vi "曲线模型计算.vi"(11 "曲线模型":T2={"标液浓度1"=0.0, "测量吸光度1"=0.0, "样品1启用"=FALSE, "标液浓度2"=0.0, "测量吸光度2"=0.0, "样品2启用"=FALSE, "标液浓度3"=0.0, "测量吸光度3"=0.0, "样品3启用"=FALSE, "标液浓度4"=0.0, "测量吸光度4"=0.0, "样品4启用"=FALSE, "标液浓度5"=0.0, "测量吸光度5"=0.0, "样品5启用"=FALSE, "模型"=enum."线性", "精度"=4.0, "XY图"=[], "拟合公式"="", "r^2"=0.0, "标样一校准时间"=timestamp(0 s since 1904-01-01), "标样二校准时间"=timestamp(0 s since 1904-01-01), "标样三校准时间"=timestamp(0 s since 1904-01-01), "标样四校准时间"=timestamp(0 s since 1904-01-01), "标样五校准时间"=timestamp(0 s since 1904-01-01), "二次方程"={"x^2"=0.0, "K"=0.0, "B"=0.0}, "标定时间"=timestamp(0 s since 1904-01-01), "拟合公式 2"="", "r^2 2"=0.0} {"r^2 2" format="%.7f"; "标定时间" format="%<%Y/%m/%d %H:%M:%S>T"; "标样五校准时间" format="%<%Y/%m/%d %H:%M:%S>T"; "标样四校准时间" format="%<%Y/%m/%d %H:%M:%S>T"; "标样三校准时间" format="%<%Y/%m/%d %H:%M:%S>T"; "标样二校准时间" format="%<%Y/%m/%d %H:%M:%S>T"; "标样一校准时间" format="%<%Y/%m/%d %H:%M:%S>T"; "r^2" format="%.7f"; "测量吸光度5" format="%#.6f"; "测量吸光度4" format="%#.6f"; "测量吸光度3" format="%#.6f"; "测量吸光度2" format="%#.6f"; "测量吸光度1" format="%#.6f"}) -> (1 "公式切换阈值滴定数(0~9999)":dbl, 2 "二次方程 2":cluster{"K":dbl, "B":dbl, "x^2":dbl}, 3 "输出簇":T1)   [LabVIEW 2016, in "斯坦道CODMn.lvlib"]
uses:
  <vilib>/Analysis/6fits.llb/Curve Fitting Criteria.ctl
  <vilib>/Analysis/NI_AALPro.lvlib
panel:
  # "校准时间"
  # "标液浓度"
  # "滴定数"
  # "标液一"
  # "标液二"
  # "标液三"
  # "零点"
  # "跨度"
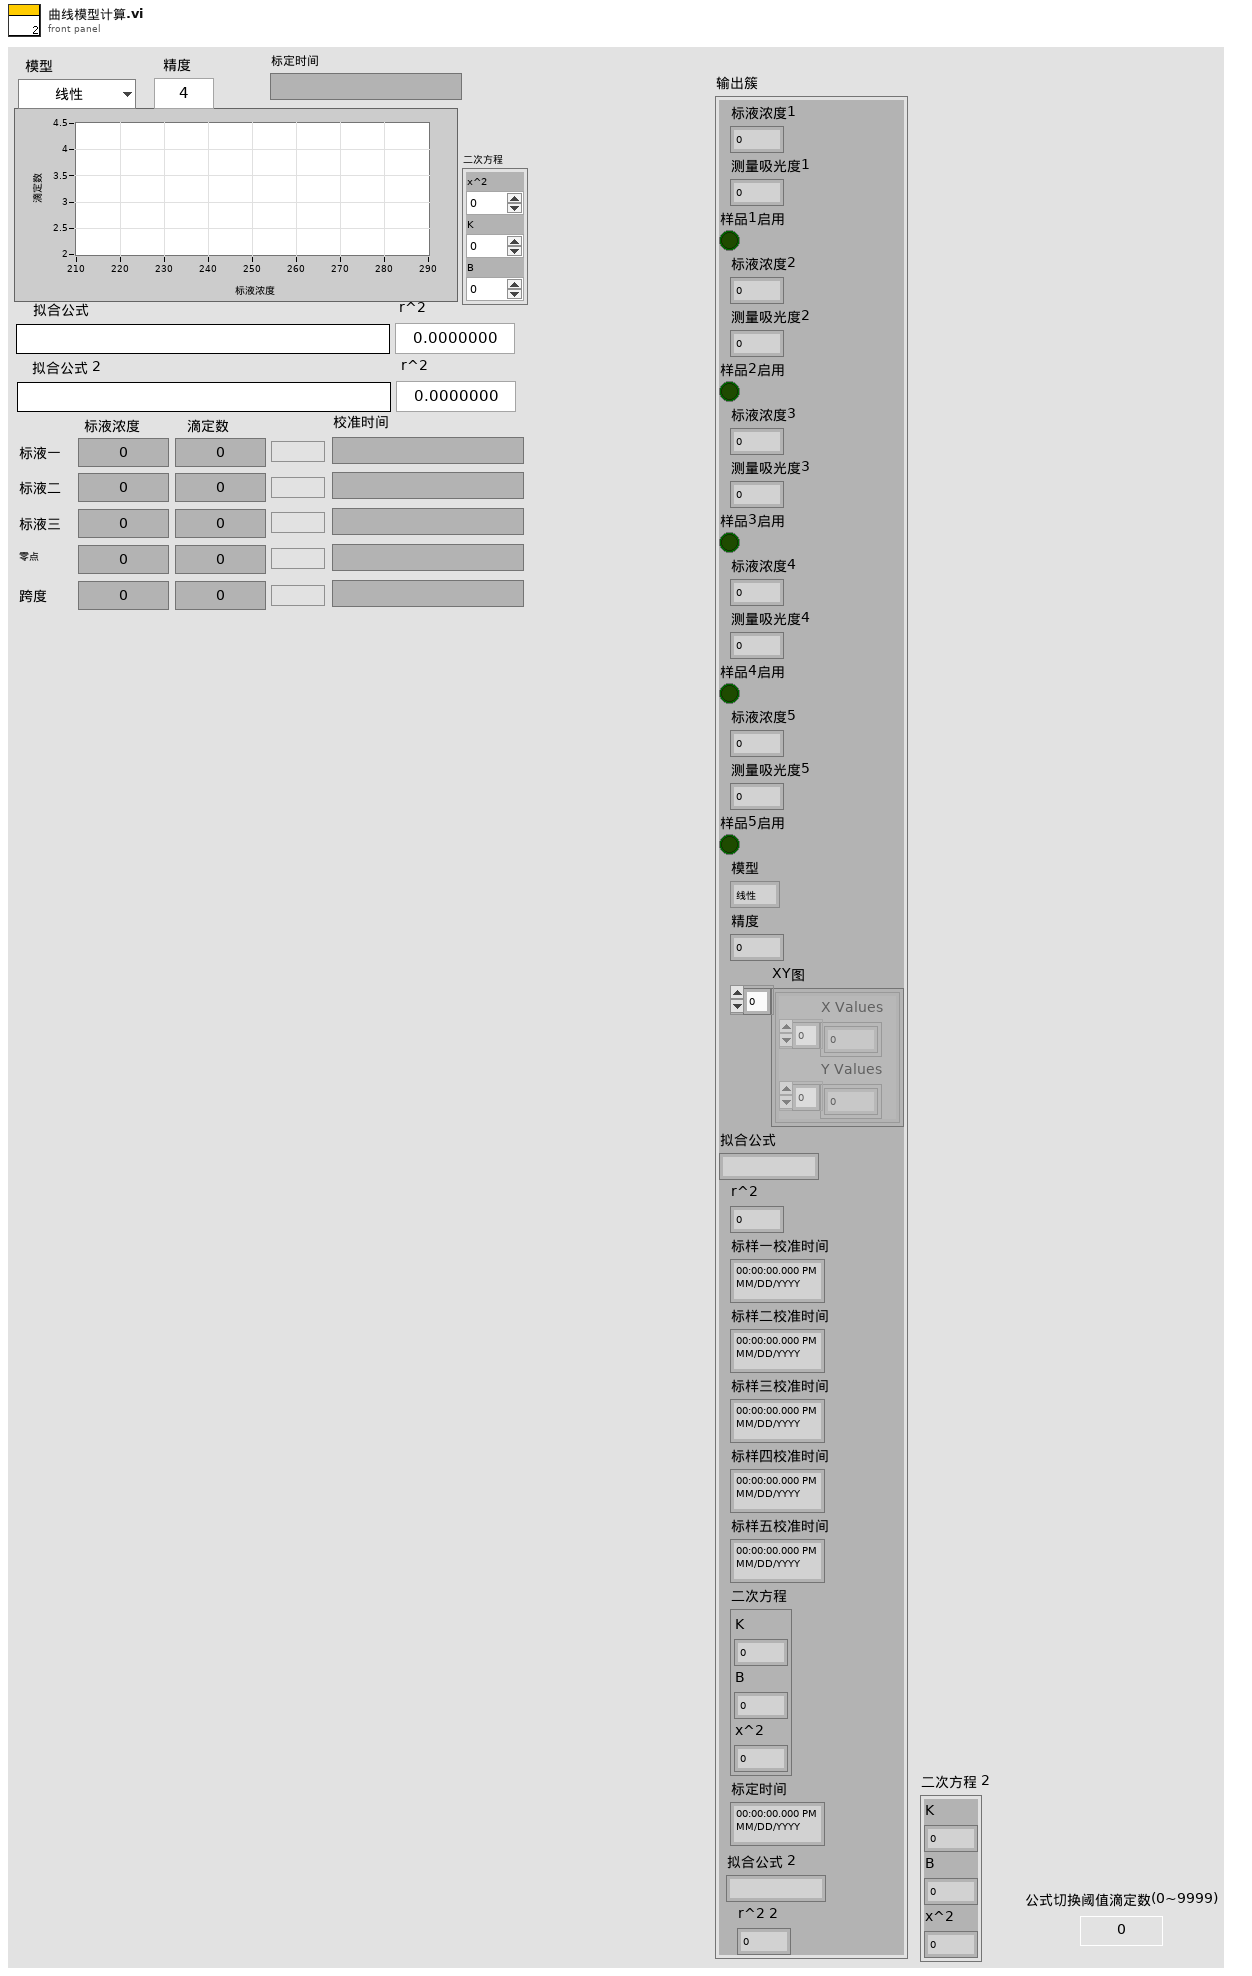
[diagram p1: front panel]
types:
  T1 = cluster{"标液浓度1":dbl, "测量吸光度1":dbl, "样品1启用":bool, "标液浓度2":dbl, "测量吸光度2":dbl, "样品2启用":bool, "标液浓度3":dbl, "测量吸光度3":dbl, "样品3启用":bool, "标液浓度4":dbl, "测量吸光度4":dbl, "样品4启用":bool, "标液浓度5":dbl, "测量吸光度5":dbl, "样品5启用":bool, "模型":enum32{"线性", "多项式", "折线"}, "精度":dbl, "XY图":cluster{"X Values":dbl[], "Y Values":dbl[]}[], "拟合公式":string, "r^2":dbl, "标样一校准时间":timestamp, "标样二校准时间":timestamp, "标样三校准时间":timestamp, "标样四校准时间":timestamp, "标样五校准时间":timestamp, "二次方程":cluster{"c":dbl, "B":dbl, "x^2":dbl}, "标定时间":timestamp, "拟合公式 2":string, "r^2 2":dbl}
  T2 = cluster{"标液浓度1":dbl, "测量吸光度1":dbl, "样品1启用":bool, "标液浓度2":dbl, "测量吸光度2":dbl, "样品2启用":bool, "标液浓度3":dbl, "测量吸光度3":dbl, "样品3启用":bool, "标液浓度4":dbl, "测量吸光度4":dbl, "样品4启用":bool, "标液浓度5":dbl, "测量吸光度5":dbl, "样品5启用":bool, "模型":enum32{"线性", "多项式", "折线"}, "精度":dbl, "XY图":cluster{"X Values":dbl[], "Y Values":dbl[]}[], "拟合公式":string, "r^2":dbl, "标样一校准时间":timestamp, "标样二校准时间":timestamp, "标样三校准时间":timestamp, "标样四校准时间":timestamp, "标样五校准时间":timestamp, "二次方程":cluster{"x^2":dbl, "K":dbl, "B":dbl}, "标定时间":timestamp, "拟合公式 2":string, "r^2 2":dbl}
  T3 = typedef "NI_AALPro.lvlib/Curve Fitting Criteria.ctl" = u16
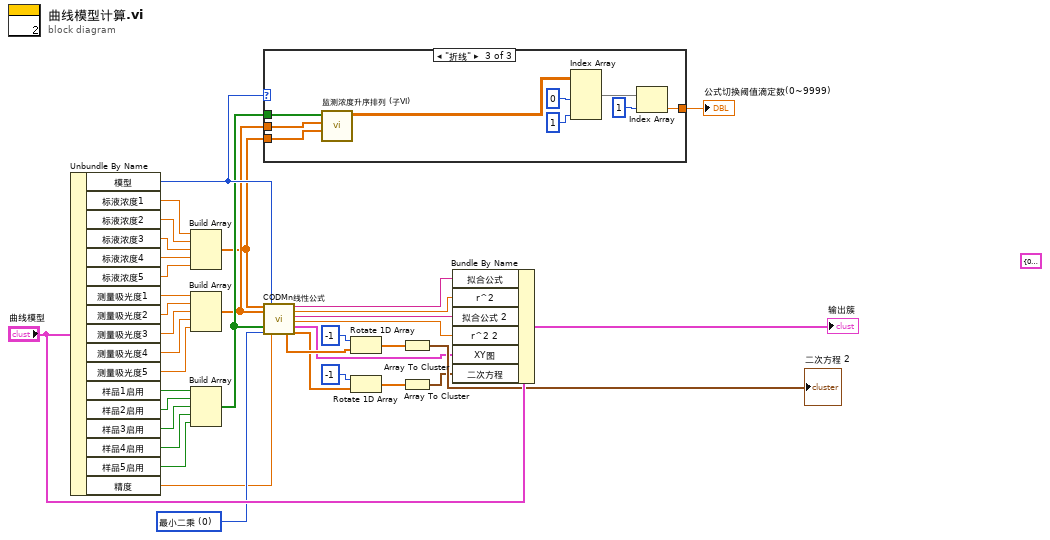
[diagram p0: block diagram]
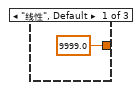
[diagram p2: hidden frame]
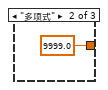
[diagram p3: hidden frame]
diagram:
  (unwired) T1 {"标液浓度1"=0.0, "测量吸光度1"=0.0, "样品1启用"=FALSE, "标液浓度2"=0.0, "测量吸光度2"=0.0, "样品2启用"=FALSE, "标液浓度3"=0.0, "测量吸光度3"=0.0, "样品3启用"=FALSE, "标液浓度4"=0.0, "测量吸光度4"=0.0, "样品4启用"=FALSE, "标液浓度5"=0.0, "测量吸光度5"=0.0, "样品5启用"=FALSE, "模型"=enum."线性", "精度"=0.0, "XY图"=[], "拟合公式"="", "r^2"=0.0, "标样一校准时间"=timestamp(0 s since 1904-01-01), "标样二校准时间"=timestamp(0 s since 1904-01-01), "标样三校准时间"=timestamp(0 s since 1904-01-01), "标样四校准时间"=timestamp(0 s since 1904-01-01), "标样五校准时间"=timestamp(0 s since 1904-01-01), "二次方程"={"c"=0.0, "B"=0.0, "x^2"=0.0}, "标定时间"=timestamp(0 s since 1904-01-01), "拟合公式 2"="", "r^2 2"=0.0} ("输出簇")
  w18 = T3 0 items=["最小二乘", "最小绝对残差", "Bisquare"] ("method")
  n1 = Unbundle By Name("曲线模型") -> ("模型"=w19:enum32{"线性", "多项式", "折线"}, "标液浓度1"=w37:dbl, "标液浓度2"=w36:dbl, "标液浓度3"=w35:dbl, "标液浓度4"=w34:dbl, "标液浓度5"=w33:dbl, "测量吸光度1"=w32:dbl, "测量吸光度2"=w31:dbl, "测量吸光度3"=w30:dbl, "测量吸光度4"=w29:dbl, "测量吸光度5"=w28:dbl, "样品1启用"=w27:bool, "样品2启用"=w26:bool, "样品3启用"=w25:bool, "样品4启用"=w24:bool, "样品5启用"=w23:bool, "精度"=w17:dbl)
  n2 = Build Array(w37, w36, w35, w34, w33) -> (w1:dbl[])
  n3 = Build Array(w32, w31, w30, w29, w28) -> (w2:dbl[])
  n4 = Build Array(w27, w26, w25, w24, w23) -> (w3:bool[])
  n5 = case shown="\"折线\"" w19 {
    tunnel: [9999.0 ("数值") 9999.0 ("数值") w44] -> w20
    tunnel: w3 -> [_ _ w43]
    tunnel: w2 -> [_ _ w42]
    tunnel: w1 -> [_ _ w41]
    frame "线性", Default {
    }
    frame "多项式" {
    }
    frame "折线" {
      n6 = call "监测浓度升序排列 (子VI).vi"("标液浓度"=w41, "滴定数"=w42, "启用"=w43) -> ("输出数组"=w40:dbl[][])  [unwired: 8 in]
      n7 = Index Array(array=w40, index (col) #1=0 ("禁用的索引 (列)"), index (col) #2=1 ("索引 (列)")) -> (element #1=w45:dbl[])  [unwired: 2 in, 1 out]
      n8 = Index Array(array=w45, index=1 ("索引")) -> (element=w44:dbl)
    }
  }
  "公式切换阈值滴定数(0~9999)" <- w20
  n9 = call "CODMn线性公式.vi"("标液浓度"=w1, "滴定数"=w2, "启用"=w3, "method"=w18, "模型"=w19, "精度"=w17) -> ("Polynomial Coefficients 2"=w13:dbl[], "拟合方程"=w4:string, "r^2"=w5:dbl, "拟合方程 2"=w6:string, "r^2 2"=w7:dbl, "XY图"=w8:cluster{"X Values":dbl[], "Y Values":dbl[]}[], "Polynomial Coefficients"=w10:dbl[])  [unwired: 7 in]
  n10 = Rotate 1D Array(1:w13, 2:-1 ("n")) -> (0:w16:dbl[])
  n11 = Rotate 1D Array(1:w10, 2:-1 ("n")) -> (0:w12:dbl[])
  n12 = Array To Cluster(array=w16) -> (cluster=→"二次方程 2":cluster{"[0]":dbl, "[1]":dbl, "[2]":dbl})
  n13 = Array To Cluster(array=w12) -> (cluster=w9:cluster{"[0]":dbl, "[1]":dbl, "[2]":dbl})
  n14 = Bundle By Name(cluster="曲线模型", "拟合公式"=w4, "r^2"=w5, "拟合公式 2"=w6, "r^2 2"=w7, "XY图"=w8, "二次方程"=w9) -> (→"输出簇":T2)
